vi "wyjscia joya.vi"(9 "index joya jazda":i32=2) -> (0 "error out":errorcluster, 1 "wyjscia joya":T3, 2 "axis info":T4, 3 "Refnum out":refnum<k1>)   [LabVIEW 2014]
uses:
  Wyjscia joya.ctl
  <vilib>/Utility/inputDevices.llb/joystickAcquire.vi
panel:
  out "direction info":T1
  out "button info":T2
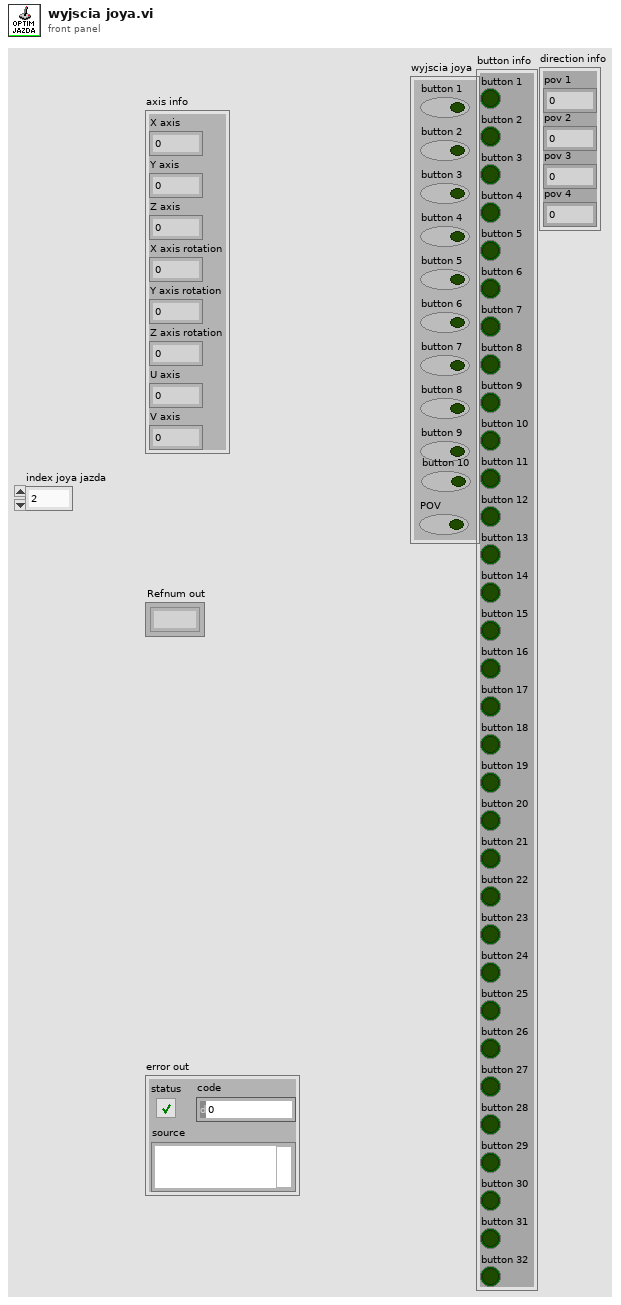
[diagram p1: front panel]
types:
  T1 = cluster{"pov 1":i32, "pov 2":i32, "pov 3":i32, "pov 4":i32}
  T2 = cluster{"button 1":bool, "button 2":bool, "button 3":bool, "button 4":bool, "button 5":bool, "button 6":bool, "button 7":bool, "button 8":bool, "button 9":bool, "button 10":bool, "button 11":bool, "button 12":bool, "button 13":bool, "button 14":bool, "button 15":bool, "button 16":bool, "button 17":bool, "button 18":bool, "button 19":bool, "button 20":bool, "button 21":bool, "button 22":bool, "button 23":bool, "button 24":bool, "button 25":bool, "button 26":bool, "button 27":bool, "button 28":bool, "button 29":bool, "button 30":bool, "button 31":bool, "button 32":bool}
  T3 = typedef "Wyjscia joya.ctl" = cluster{"button 1":bool, "button 2":bool, "button 3":bool, "button 4":bool, "button 5":bool, "button 6":bool, "button 7":bool, "button 8":bool, "button 9":bool, "POV":bool, "button 10":bool}
  T4 = cluster{"X axis":i32, "Y axis":i32, "Z axis":i32, "X axis rotation":i32, "Y axis rotation":i32, "Z axis rotation":i32, "U axis":i32, "V axis":i32}
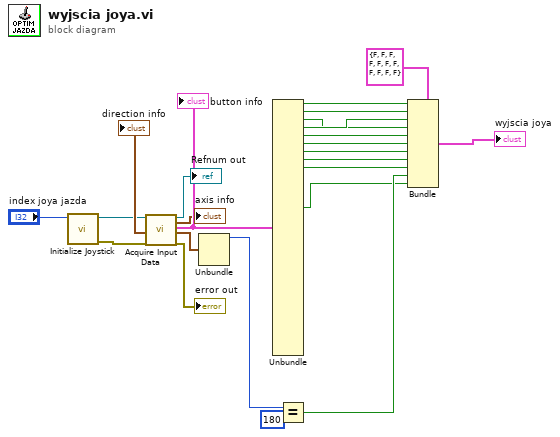
[diagram p0: block diagram]
diagram:
  n1 = call <vilib>:"Initialize Joystick.vi"("device index"="index joya jazda") -> ("error out"=w6:errorcluster, "device ID"=w7:refnum<k1>)  [unwired: 9 in]
  n2 = call-poly <vilib>:"Acquire Input Data.vi"("device ID"=w7, "error in (no error)"=w6) -> ("device ID"=→"Refnum out":refnum<k1>, "axis info"=→"axis info":T4, "button info"=w21:T2, "direction info"=w23:T1, "error out"=→"error out":errorcluster)  [unwired: 13 in]
  "button info" <- w21
  "direction info" <- w23
  n3 = Unbundle(w23) -> ("pov 1"=w3:i32)  [unwired: 3 out]
  n4 = Unbundle(w21) -> ("button 1"=w5:bool, "button 2"=w17:bool, "button 3"=w1:bool, "button 4"=w2:bool, "button 5"=w16:bool, "button 6"=w15:bool, "button 7"=w14:bool, "button 8"=w13:bool, "button 9"=w12:bool, "button 14"=w4:bool)  [unwired: 22 out]
  n5 = Equal?(x=w3, y=180) -> (x = y?=w11:bool)
  n6 = Bundle(cluster=T3 {"button 1"=FALSE, "button 2"=FALSE, "button 3"=FALSE, "button 4"=FALSE, "button 5"=FALSE, "button 6"=FALSE, "button 7"=FALSE, "button 8"=FALSE, "button 9"=FALSE, "POV"=FALSE, "button 10"=FALSE}, "button 1"=w5, "button 2"=w17, "button 3"=w2, "button 4"=w1, "button 5"=w16, "button 6"=w15, "button 7"=w14, "button 8"=w13, "button 9"=w12, "POV"=w11, "button 10"=w4) -> (→"wyjscia joya":T3)
